vi "ErrorMessages1.vi"(8 "source":string="Custom Message", 10 "code":i32=5000) -> (0 "Error Out":errorcluster)   [LabVIEW 2016]
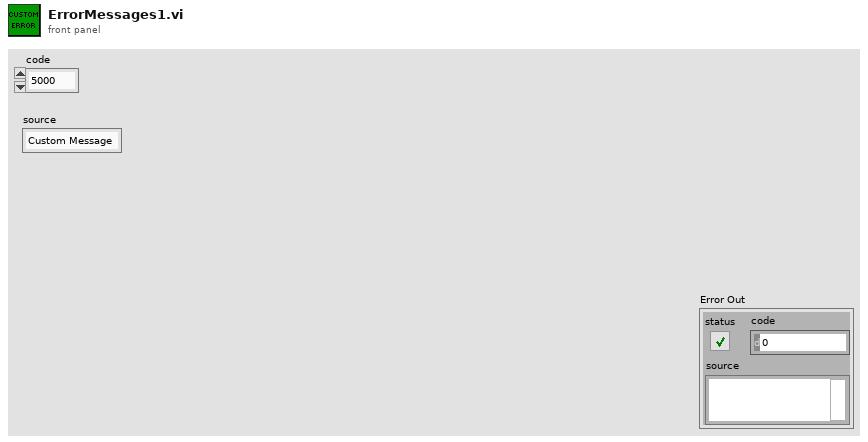
[diagram p1: front panel]
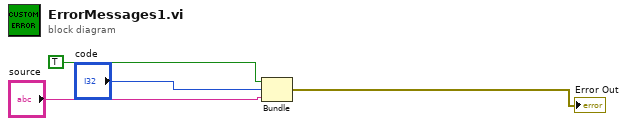
[diagram p0: block diagram]
diagram:
  n1 = Bundle("status"=TRUE, "code"="code", "source"="source") -> (→"Error Out":errorcluster)  [unwired: 1 in]
